vi "Cockpit UDP sender v2.vi"() -> ()   [LabVIEW 2010]
panel:
  in  "right_pedal":bool
  in  "left_pedal":bool
  in  "up_pedal":bool
  in  "gripper":sgl
  in  "down_pedal":sgl format="%.2f"
  in  "enc 4":sgl
  in  "enc 3":sgl
  in  "enc 2":sgl
  in  "enc 1":sgl
  in  "stop":bool
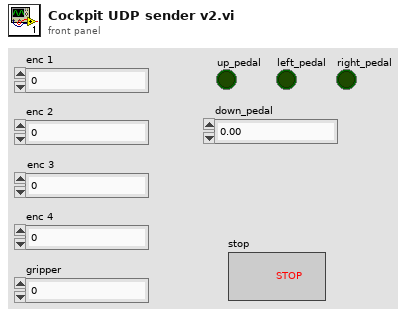
[diagram p1: front panel]
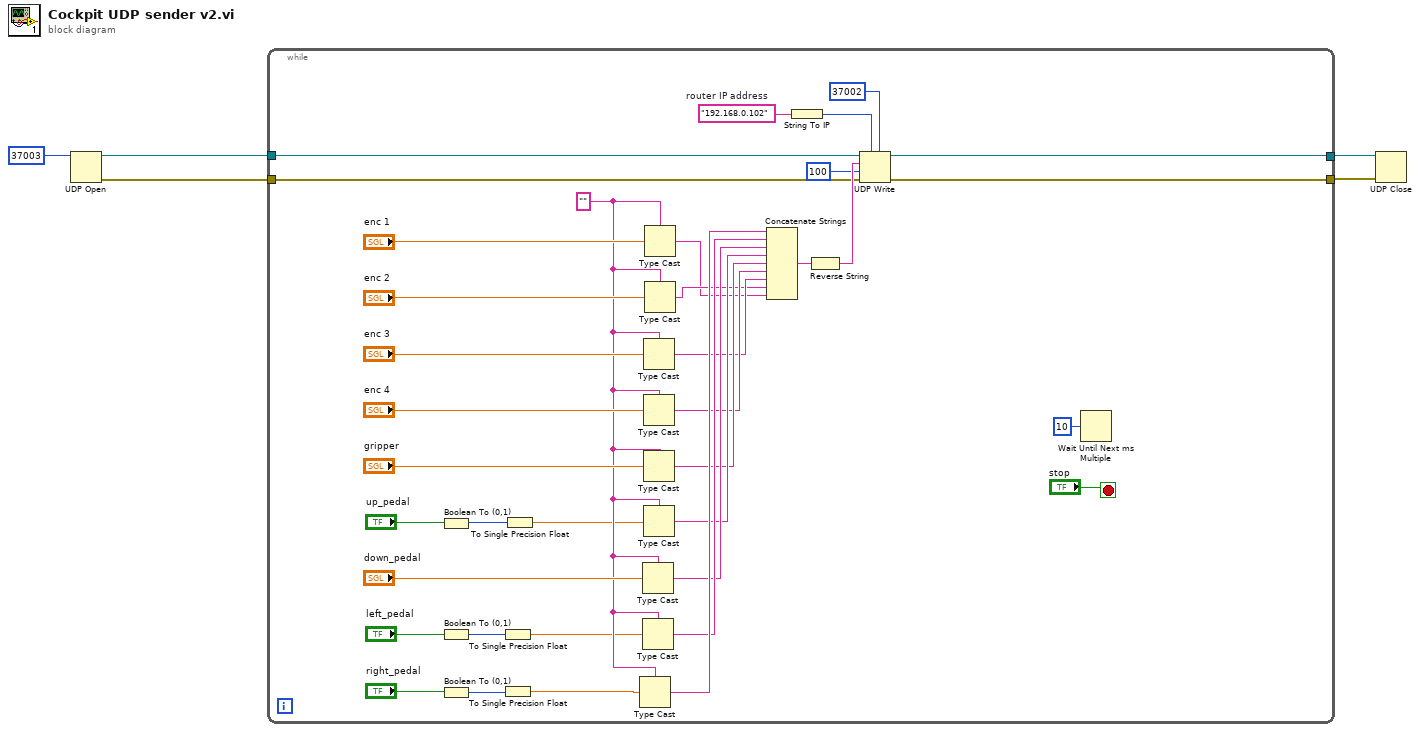
[diagram p0: block diagram]
diagram:
  n1 = UDP Open(11:u16 37003 ("port")) -> (port=w4:refnum<k16>, 0:w2:errorcluster)  [unwired: 4 in, 1 out]
  n2 = while {
    tunnel: w4 -> [w36]
    tunnel: [w41] -> w3
    tunnel: w2 -> [w35]
    tunnel: [w40] -> w1
    stop <- "stop" stop-if-true
    w8 = "192.168.0.102"  # router IP address
    w25 = "" ("reversed")
    n3 = Boolean To (0,1)(Boolean="up_pedal") -> (0, 1=w15:i16)
    n4 = Boolean To (0,1)(Boolean="left_pedal") -> (0, 1=w11:i16)
    n5 = Boolean To (0,1)(Boolean="right_pedal") -> (0, 1=w13:i16)
    n6 = To Single Precision Float(number=w11) -> (single precision float=w10:sgl)
    n7 = To Single Precision Float(number=w13) -> (single precision float=w12:sgl)
    n8 = To Single Precision Float(number=w15) -> (single precision float=w14:sgl)
    n9 = Type Cast(type=w25, x=w12) -> (*(type *) &x=w24:string)
    n10 = Type Cast(type=w25, x="down_pedal") -> (*(type *) &x=w22:string)
    n11 = Type Cast(type=w25, x=w10) -> (*(type *) &x=w23:string)
    n12 = Type Cast(type=w25, x="enc 3") -> (*(type *) &x=w18:string)
    n13 = Type Cast(type=w25, x="enc 4") -> (*(type *) &x=w19:string)
    n14 = Type Cast(type=w25, x="gripper") -> (*(type *) &x=w20:string)
    n15 = Type Cast(type=w25, x=w14) -> (*(type *) &x=w21:string)
    n16 = Type Cast(type=w25, x="enc 1") -> (*(type *) &x=w16:string)
    n17 = Type Cast(type=w25, x="enc 2") -> (*(type *) &x=w17:string)
    n18 = Concatenate Strings(w24, w23, w22, w21, w20, w19, w18, w17, w16) -> (w39:string)
    n19 = String To IP(1:w8) -> (0:w7:u32)
    n20 = Reverse String(1:w39) -> (0:w38:string)
    n21 = UDP Write(address=w7, port or service name=u16 37002, connection ID=w36, data in=w38, 8:w35, 9:100 ("timeout ms (25000)")) -> (error out=w40:errorcluster, 3:w41:refnum<k16>)
    n22 = Wait Until Next ms Multiple(millisecond multiple=u32 10) -> ()  [unwired: 1 out]
  }
  n23 = UDP Close(connection ID=w3, 8:w1) -> ()  [unwired: 2 out]
